vi "Comm Connect.vi"(8 "error in (no error)":errorcluster, 11 "niDTS Comm Telnet in":refnum<class "niDTS Comm Telnet.lvclass">) -> (0 "error out":errorcluster, 3 "niDTS Comm Telnet out":refnum<class "niDTS Comm Telnet.lvclass">)   [LabVIEW 2015, in "niDTS CommLib.lvlib" / "niDTS Comm Telnet.lvclass"]
uses:
  niDTS Comm Telnet.lvclass
  Framework/Logger/Includes/niDTS Logger INC Log Element Type.ctl
  Framework/Logger/Objects/BASE_class/niDTS Logger.lvclass
  Utility/telnet/NI_InternetTK_Core_VIs.lvlib
  Framework/niDTS Framework.lvlib
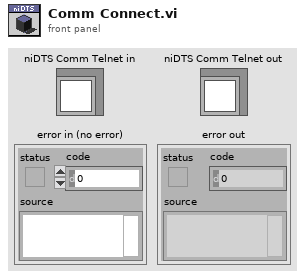
[diagram p1: front panel]
types:
  T1 = typedef "niDTS Framework.lvlib/niDTS Logger INC Log Element Type.ctl" = enum16{"Error", "Warning", "Information", "Debugging"}
  T2 = typedef "niDTS CommLib.lvlib/niDTS Comm INC Telnet Port Parameters.ctl" = cluster{"Bytes to Read":i32, "Line Separator":string, "Port Timeout (ms)":i32, "Read Mode":enum16{"normal", "line", "buffered"}, "Write Mode":enum16{"normal", "line", "buffered"}, "Remote Port":u16}
  T3 = typedef "niDTS Framework.lvlib/niDTS Logger INC Handle.ctl" = refnum<data-value>
  T4 = typedef "Telnet Session.ctl" = refnum<k1>
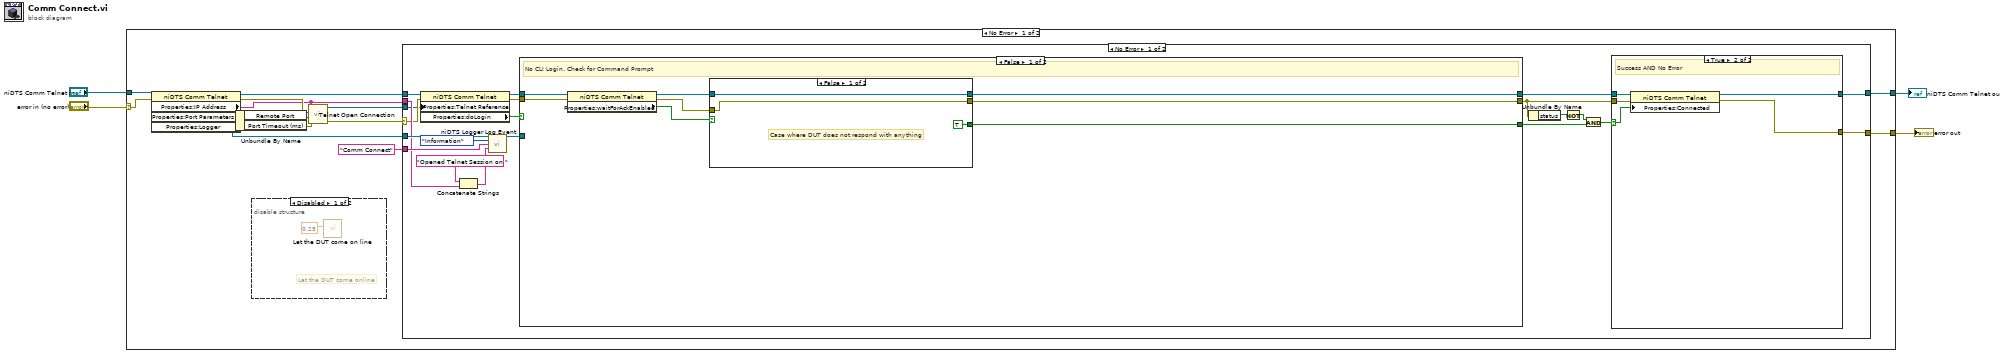
[diagram p0: block diagram]
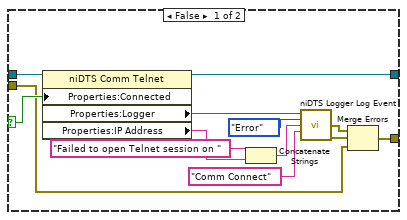
[diagram p3: hidden frame]
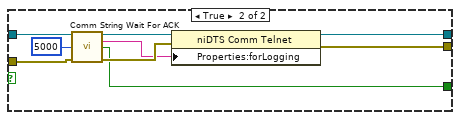
[diagram p4: hidden frame]
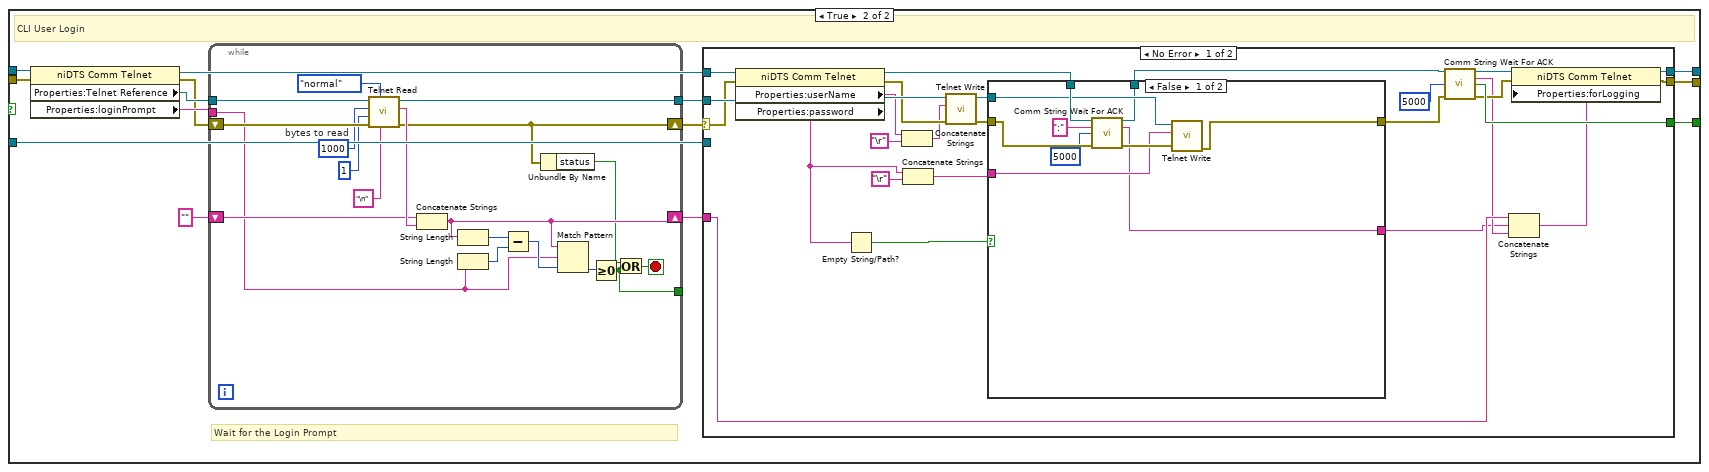
[diagram p5: hidden frame]
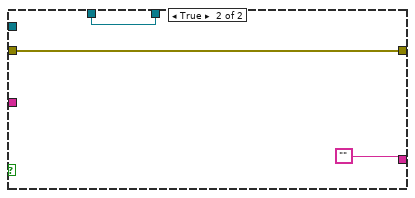
[diagram p6: hidden frame]
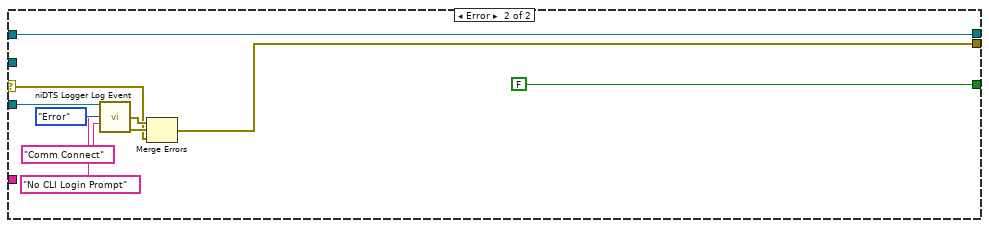
[diagram p7: hidden frame]
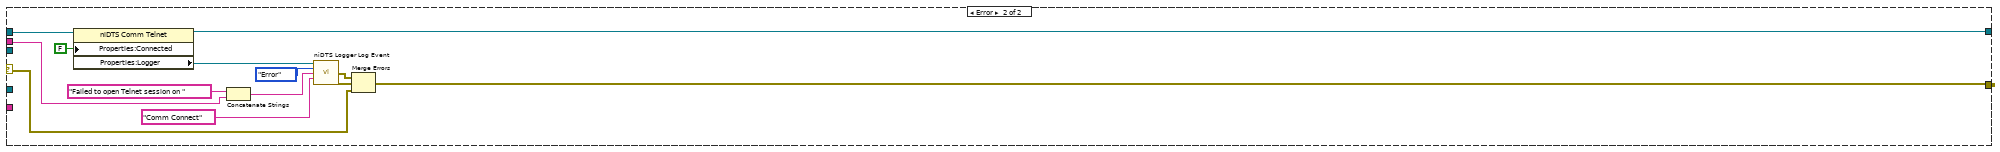
[diagram p8: hidden frame]
diagram:
  n1 = case shown="No Error" "error in (no error)" {
    selector: "error in (no error)" -> [w11 w174]
    tunnel: "niDTS Comm Telnet in" -> [w18 w175]
    tunnel: [w8 w175] -> w2
    tunnel: [w5 w174] -> w1
    frame No Error {
      n2 = property class="niDTS Comm Telnet"(reference=w18, error in=w11) -> (reference out=w10:refnum<class "niDTS Comm Telnet.lvclass">, error out=w14:errorcluster, "Properties:IP Address"=w9:string, "Properties:Port Parameters"=w17:T2, "Properties:Logger"=w7:T3)
      n3 = Unbundle By Name(w17) -> ("Remote Port"=w16:u16, "Port Timeout (ms)"=w15:i32)
      n4 = disable-structure shown="Disabled" {
        frame Disabled {
          # "Let the DUT come online"
          n5 = call "Let the DUT come on line"("Delay Time (s)"=0.25) -> ()  [unwired: 10 in, 1 out]
        }
        frame Enabled {
        }
      }
      n6 = call "Telnet Open Connection.vi"("error in (no error)"=w14, "timeout ms (60000)"=w15, "remote port (23)"=w16, "address"=w9) -> ("error out"=w13:errorcluster, "telnet connection"=w12:T4)  [unwired: 6 in]
      n7 = case shown="No Error" w13 {
        selector: w13 -> [w33 w163]
        tunnel: w12 -> [w32 _]
        tunnel: w10 -> [w34 w173]
        tunnel: w9 -> [w36 w166]
        tunnel: [w20 w162] -> w5
        tunnel: [w21 w161] -> w8
        tunnel: w7 -> [w40 _]
        tunnel: "Comm Connect" ("Description/Data") -> [w38 _]
        frame No Error {
          n8 = property class="niDTS Comm Telnet"(reference=w34, error in=w33, "Properties:Telnet Reference"=w32) -> (reference out=w30:refnum<class "niDTS Comm Telnet.lvclass">, error out=w29:errorcluster, "Properties:doLogin"=w31:bool)
          n9 = Concatenate Strings("Opened Telnet Session on ", w36) -> (w35:string)
          n10 = call "niDTS Logger Log Event.vi"("Logger Handle"=w40, "Type"=niDTS_Logger_INC_Log_Element_Type."Information", "Description/Data"=w38, "Source/Location"=w35) -> ("Logger Handle out"=w28:T3)  [unwired: 9 in, 2 out]
          n11 = case shown="False" w31 {
            tunnel: w30 -> [w61 w92]
            tunnel: w29 -> [w66 w91]
            tunnel: w28 -> [_ w83]
            tunnel: [w65 w81] -> w27
            tunnel: [w64 w80] -> w23
            tunnel: [w63 w79] -> w22
            frame False {
              # "No CLI Login. Check for Command Prompt"
              n12 = property class="niDTS Comm Telnet"(reference=w61, error in=w66) -> (reference out=w60:refnum<class "niDTS Comm Telnet.lvclass">, error out=w62:errorcluster, "Properties:waitForAckEnabled"=w59:bool)
              n13 = case shown="False" w59 {
                tunnel: w60 -> [w68 w77]
                tunnel: w62 -> [w67 w75]
                tunnel: [TRUE ("Sucess") w72] -> w65
                tunnel: [w68 w71] -> w64
                tunnel: [w67 w70] -> w63
                frame False {
                  # "Case where DUT does not respond with anything"
                }
                frame True {
                  n14 = call-dynamic "Comm String Wait For ACK.vi"("niDTS Comm Telnet in"=w77, "Timeout (ms)"=5000, "error in (no error)"=w75) -> ("niDTS Comm Telnet out"=w76:refnum<class "niDTS Comm Telnet.lvclass">, "Response"=w73:string, "Sucess"=w72:bool, "error out"=w74:errorcluster)  [unwired: 9 in]
                  n15 = property class="niDTS Comm Telnet"(reference=w76, error in=w74, "Properties:forLogging"=w73) -> (reference out=w71:refnum<class "niDTS Comm Telnet.lvclass">, error out=w70:errorcluster)
                }
              }
            }
            frame True {
              # "Wait for the Login Prompt"
              # "CLI User Login"
              n16 = property class="niDTS Comm Telnet"(reference=w92, error in=w91) -> (reference out=w84:refnum<class "niDTS Comm Telnet.lvclass">, error out=w87:errorcluster, "Properties:Telnet Reference"=w89:T4, "Properties:loginPrompt"=w88:string)
              n17 = while "Wait for the login prompt" {
                tunnel: [w148] -> w85
                shift-right: [w149] -> w82
                shift-left: "" -> [w155]
                tunnel: w89 -> [w154]
                shift-right: [w146] -> w86
                shift-left: w87 -> [w160]
                tunnel: w88 -> [w147]
                tunnel: [w142] -> _
                stop <- w144 stop-if-true
                w158 = 1000  # bytes to read
                n18 = call "Telnet Read.vi"("line separator"="\n", "read mode (normal)"=enum16{"normal", "line", "buffered"}."normal", "error in (no error)"=w160, "timeout ms (25000)"=1, "bytes to read"=w158, "telnet connection"=w154) -> ("error out"=w146:errorcluster, "data out"=w156:string, "telnet connection out"=w148:T4)  [unwired: 1 in]
                n19 = Concatenate Strings(w155, w156) -> (w149:string)
                n20 = String Length(string=w149) -> (length=w152:i32)
                n21 = String Length(string=w147) -> (length=w151:i32)
                n22 = Subtract(x=w152, y=w151) -> (x-y=w150:i32)
                n23 = Unbundle By Name(w146) -> ("status"=w145:bool)
                n24 = Match Pattern(string=w149, regular expression=w147, offset (0)=w150) -> (offset past match=w153:i32)  [unwired: 3 out]
                n25 = Greater Or Equal To 0?(x=w153) -> (x >= 0?=w142:bool)
                n26 = Or(x=w145, y=w142) -> (x .or. y?=w144:bool)
              }
              n27 = case shown="No Error" w86 {
                selector: w86 -> [w116 w133]
                tunnel: w85 -> [w118 _]
                tunnel: w84 -> [w117 w134]
                tunnel: w83 -> [_ w136]
                tunnel: [w113 FALSE ("Sucess")] -> w81
                tunnel: w82 -> [w107 _]
                tunnel: [w109 w134] -> w80
                tunnel: [w108 w132] -> w79
                frame No Error {
                  n28 = property class="niDTS Comm Telnet"(reference=w117, error in=w116) -> (reference out=w103:refnum<class "niDTS Comm Telnet.lvclass">, error out=w114:errorcluster, "Properties:userName"=w98:string, "Properties:password"=w94:string)
                  n29 = Empty String/Path?(string/path=w94) -> (empty?=w106:bool)
                  n30 = Concatenate Strings(w98, "\r") -> (w96:string)
                  n31 = Concatenate Strings(w94, "\r") -> (w93:string)
                  n32 = call "Telnet Write.vi"("error in (no error)"=w114, "data in"=w96, "telnet connection"=w118) -> ("error out"=w105:errorcluster, "telnet connection out"=w102:T4)  [unwired: 4 in, 1 out]
                  n33 = case shown="False" w106 {
                    tunnel: w105 -> [w126 w131]
                    tunnel: [w121 w131] -> w104
                    tunnel: w103 -> [w128 w130]
                    tunnel: w102 -> [w125 _]
                    tunnel: w93 -> [w123 _]
                    tunnel: [w122 w130] -> w101
                    tunnel: [w120 ""] -> w99
                    frame False {
                      n34 = call-dynamic "Comm String Wait For ACK.vi"("niDTS Comm Telnet in"=w128, "ACK"=":", "Timeout (ms)"=5000, "error in (no error)"=w126) -> ("niDTS Comm Telnet out"=w122:refnum<class "niDTS Comm Telnet.lvclass">, "Response"=w120:string, "error out"=w124:errorcluster)  [unwired: 8 in, 1 out]
                      n35 = call "Telnet Write.vi"("error in (no error)"=w124, "data in"=w123, "telnet connection"=w125) -> ("error out"=w121:errorcluster)  [unwired: 4 in, 2 out]
                    }
                    frame True {
                    }
                  }
                  n36 = call-dynamic "Comm String Wait For ACK.vi"("niDTS Comm Telnet in"=w101, "Timeout (ms)"=5000, "error in (no error)"=w104) -> ("niDTS Comm Telnet out"=w112:refnum<class "niDTS Comm Telnet.lvclass">, "Response"=w100:string, "Sucess"=w113:bool, "error out"=w111:errorcluster)  [unwired: 9 in]
                  n37 = Concatenate Strings(w107, w99, w100) -> (w110:string)
                  n38 = property class="niDTS Comm Telnet"(reference=w112, error in=w111, "Properties:forLogging"=w110) -> (reference out=w109:refnum<class "niDTS Comm Telnet.lvclass">, error out=w108:errorcluster)
                }
                frame Error {
                  n39 = call "niDTS Logger Log Event.vi"("Logger Handle"=w136, "Type"=niDTS_Logger_INC_Log_Element_Type."Error", "Description/Data"="No CLI Login Prompt", "Source/Location"="Comm Connect" ("Description/Data")) -> ("Source Data Error"=w139:errorcluster, "error out"=w140:errorcluster)  [unwired: 9 in, 1 out]
                  n40 = Merge Errors(w139, w140, w133) -> (w132:errorcluster)
                }
              }
            }
          }
          n41 = Unbundle By Name(w22) -> ("status"=w25:bool)
          n42 = Not(x=w25) -> (.not. x?=w26:bool)
          n43 = And(x=w26, y=w27) -> (x .and. y?=w24:bool)
          n44 = case shown="True" w24 {
            selector: w24 -> [w52 w56]
            tunnel: w23 -> [w53 w58]
            tunnel: w22 -> [w43 w57]
            tunnel: [w42 w55] -> w21
            tunnel: [w41 w54] -> w20
            frame False {
              n45 = property class="niDTS Comm Telnet"(reference=w53, "Properties:Connected"=w52) -> (reference out=w42:refnum<class "niDTS Comm Telnet.lvclass">, "Properties:Logger"=w45:T3, "Properties:IP Address"=w44:string)  [unwired: 1 in, 1 out]
              n46 = Concatenate Strings("Failed to open Telnet session on " ("string"), w44) -> (w49:string)
              n47 = call "niDTS Logger Log Event.vi"("Logger Handle"=w45, "Type"=niDTS_Logger_INC_Log_Element_Type."Error", "Description/Data"=w49, "Source/Location"="Comm Connect") -> ("Source Data Error"=w48:errorcluster, "error out"=w47:errorcluster)  [unwired: 9 in, 1 out]
              n48 = Merge Errors(w48, w47, w43) -> (w41:errorcluster)
            }
            frame True {
              # "Success AND No Error"
              n49 = property class="niDTS Comm Telnet"(reference=w58, error in=w57, "Properties:Connected"=w56) -> (reference out=w55:refnum<class "niDTS Comm Telnet.lvclass">, error out=w54:errorcluster)
            }
          }
        }
        frame Error {
          n50 = property class="niDTS Comm Telnet"(reference=w173, "Properties:Connected"=FALSE ("Connected")) -> (reference out=w161:refnum<class "niDTS Comm Telnet.lvclass">, "Properties:Logger"=w168:T3)  [unwired: 1 in, 1 out]
          n51 = Concatenate Strings("Failed to open Telnet session on " ("string"), w166) -> (w165:string)
          n52 = call "niDTS Logger Log Event.vi"("Logger Handle"=w168, "Type"=niDTS_Logger_INC_Log_Element_Type."Error", "Description/Data"=w165, "Source/Location"="Comm Connect") -> ("Source Data Error"=w169:errorcluster, "error out"=w170:errorcluster)  [unwired: 9 in, 1 out]
          n53 = Merge Errors(w169, w170, w163) -> (w162:errorcluster)
        }
      }
    }
    frame Error {
    }
  }
  "error out" <- w1
  "niDTS Comm Telnet out" <- w2
